vi "Read Format Converter Configuration.vi"(8 "error in (no error)":errorcluster, 11 "Format Converter in":refnum<class "Format Converter.lvclass">) -> (0 "error out":errorcluster, 2 "Configuration":T1={"New start time"=nan, "New end time"=nan, "Output file format"=enum."ASCII", "Save ASCII column names"=TRUE, "Prepend binary array size"=FALSE, "buffer size (-1: all)"=100000, "Channels"=[], "Group"="p", "New dt"=nan} {"buffer size (-1: all)" format="%.0p"; "New start time" format="%#_10p"}, 3 "Format Converter out":refnum<class "Format Converter.lvclass">)   [LabVIEW 2018, in "Format Converter.lvclass"]
uses:
  Format Converter.lvclass
  C:/github/LabActor/Template Module/Template Module.lvclass
  NHMFL_Core/Libraries/File/File Format Converter/Format Converter Configuration.ctl
  Template Module/Template Module.lvclass/Template Module.ctl
  Template Module/Read Configuration.vi
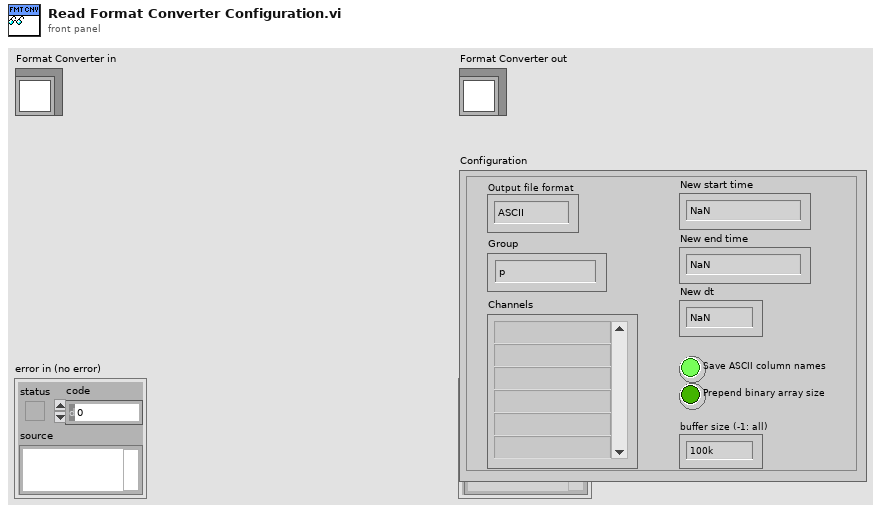
[diagram p1: front panel]
types:
  T1 = typedef "Format Converter Configuration.ctl" = cluster{"New start time":dbl, "New end time":dbl, "Output file format":enum16{"ASCII", "BINARY", "TDMS"}, "Save ASCII column names":bool, "Prepend binary array size":bool, "buffer size (-1: all)":i64, "Channels":string[], "Group":string, "New dt":dbl}
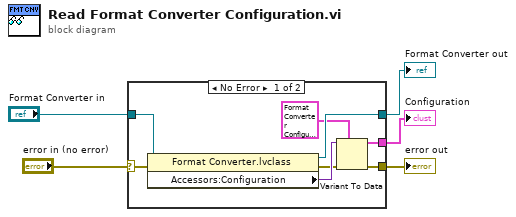
[diagram p0: block diagram]
diagram:
  n1 = case shown="No Error" "error in (no error)" {
    selector: "error in (no error)" -> [w6 w14]
    tunnel: [w11 w14] -> w4
    tunnel: [w12 w15] -> w2
    tunnel: "Format Converter in" -> [w13 w15]
    tunnel: [w8 _] -> w1
    frame No Error {
      n2 = property class="Format Converter.lvclass"(reference=w13, error in=w6) -> (reference out=w12:refnum<class "Format Converter.lvclass">, error out=w7:errorcluster, "Accessors:Configuration"=w9:variant)
      n3 = Variant To Data(error in=w7, type=T1 {"New start time"=nan, "New end time"=nan, "Output file format"=enum."ASCII", "Save ASCII column names"=TRUE, "Prepend binary array size"=FALSE, "buffer size (-1: all)"=100000, "Channels"=[], "Group"="p", "New dt"=nan} ("Format Converter Configuration"), Variant=w9) -> (data=w8:T1, error out=w11:errorcluster)
    }
    frame Error {
    }
  }
  "error out" <- w4
  "Format Converter out" <- w2
  "Configuration" <- w1
